vi "Receive Message.vi"(6 "timeout in ms (-1)":i32=-1, 8 "error in":errorcluster, 11 "NotifierMessageTransport in":refnum<class "NotifierMessageTransport.lvclass">) -> (0 "error out":errorcluster, 2 "Notifier":refnum<class "IMessagePayload.lvclass">, 3 "NotifierMessageTransport out":refnum<class "NotifierMessageTransport.lvclass">)   [LabVIEW 2016, in "NotifierMessageTransport.lvclass"]
uses:
  NotifierMessageTransport.lvclass
  IMessagePayload/IMessagePayload.lvclass
  QMHMessagePayload/QMHMessagePayload.lvclass
panel:
  # "INPUTS"
  # "OUTPUTS"
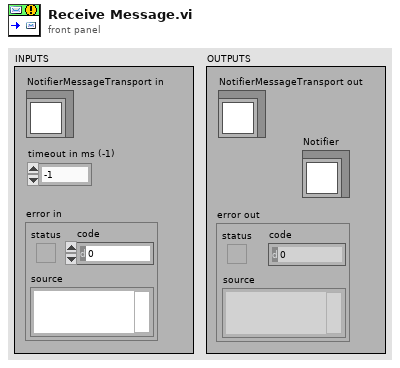
[diagram p1: front panel]
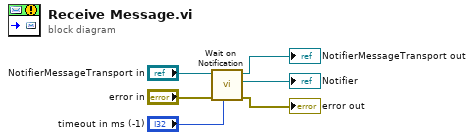
[diagram p0: block diagram]
diagram:
  n1 = call "Wait on Notification.vi"("timeout in ms (-1)"="timeout in ms (-1)", "error in"="error in", "NotifierMessageTransport in"="NotifierMessageTransport in") -> ("error out"=→"error out":errorcluster, "Notification"=→"Notifier":refnum<class "IMessagePayload.lvclass">, "NotifierMessageTransport out"=→"NotifierMessageTransport out":refnum<class "NotifierMessageTransport.lvclass">)  [unwired: 6 in]
